vi "Write Name.vi"(10 "Name":string, 11 "Network Stream in":refnum<class "Network Stream.lvclass">) -> (3 "Network Stream out":refnum<class "Network Stream.lvclass">)   [LabVIEW 2020, in "Network Stream.lvclass"]
doc: "Use this VI to specify the name of this endpoint of the network stream."
uses:
  Network Stream.lvclass
  Network Stream.lvclass/Network Stream.ctl
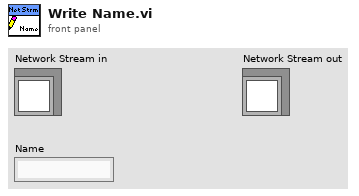
[diagram p1: front panel]
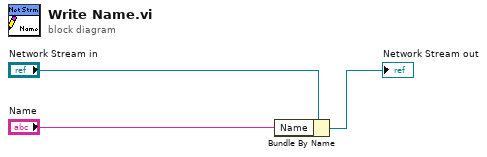
[diagram p0: block diagram]
diagram:
  n1 = Bundle By Name(cluster="Network Stream in", "Name"="Name") -> (→"Network Stream out":refnum<class "Network Stream.lvclass">)
